vi "Protocol.Convert Rate to ms Wait.vi"(11 "Rate":u32) -> (3 "ms":u32)   [LabVIEW 2015, in "J1939 Addon Engine.lvlib"]
uses:
  J1939 Addon Engine.lvlib
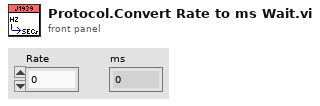
[diagram p1: front panel]
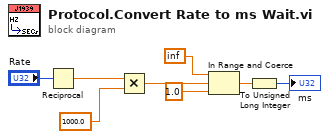
[diagram p0: block diagram]
diagram:
  n1 = Reciprocal(x="Rate") -> (1/x=w1:dbl)
  n2 = Multiply(x=w1, y=1000.0) -> (x*y=w4:dbl)
  n3 = In Range and Coerce(upper limit=inf, x=w4, lower limit=1.0) -> (coerced(x)=w5:dbl)  [unwired: 1 out]
  n4 = To Unsigned Long Integer(number=w5) -> (unsigned 32bit integer=→"ms":u32)
